vi "XML_MatchLabel.vi"(8 "error in (no error)":errorcluster caption="错误输入（无错误）", 11 "String":string) -> (0 "error out":errorcluster caption="错误输出", 3 "keyValues":T1(array[cluster]))   [LabVIEW 2014]
uses:
  <vilib>/regexp/Match Regular Expression.xnode
panel:
  out "Array":string[](array[string])
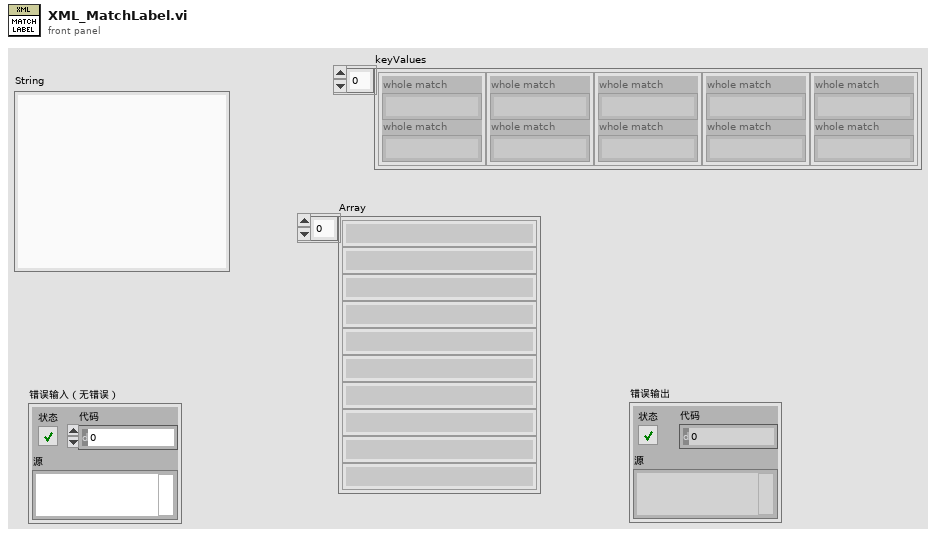
[diagram p1: front panel]
types:
  T1 = cluster{"whole match":string, "whole match":string}[]
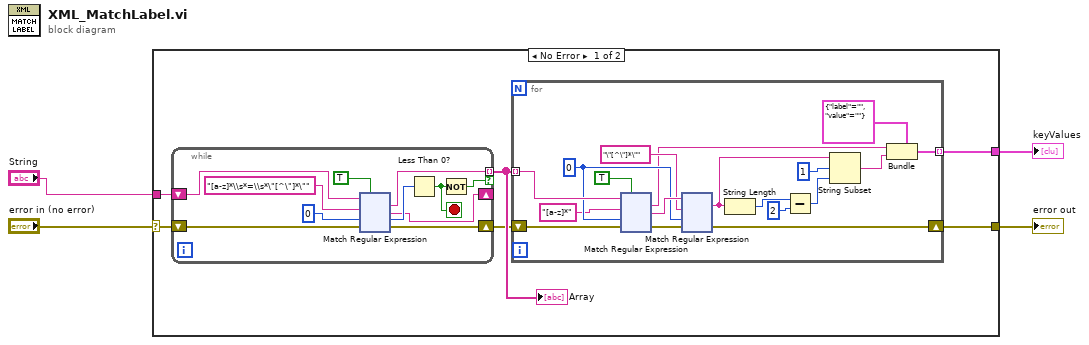
[diagram p0: block diagram]
diagram:
  n1 = case shown="No Error" "error in (no error)" {
    selector: "error in (no error)" -> [w5 w382]
    tunnel: "String" -> [w10 _]
    tunnel: [w7 w382] -> w3
    tunnel: [w6 _] -> w2
    frame No Error {
      n2 = while {
        shift-right: [w262] -> _
        shift-left: w10 -> [w267]
        tunnel: [w264] -> w9 mode=indexing if=w257
        shift-right: [w259] -> w8
        shift-left: w5 -> [w260]
        stop <- w258 stop-if-true
        n3 = xnode "Match Regular Expression"("input string"=w267, "regular expression"="[a-z]*\\s*=\\s*\"[^\"]*\"", "offset (0)"=0, "error in"=w260, "ignore case? (F)"=TRUE) -> ("whole match"=w264:string, "after match"=w262:string, "offset past match"=w263:i32, "error out"=w259:errorcluster)  [unwired: 1 in, 1 out]
        n4 = Less Than 0?(x=w263) -> (x < 0?=w258:bool)
        n5 = Not(x=w258) -> (.not. x?=w257:bool)
      }
      "Array" <- w9
      n6 = for {
        tunnel: w9 -> [w28] mode=indexing
        shift-right: [w20] -> w7
        shift-left: w8 -> [w22]
        tunnel: [w12] -> w6 mode=indexing
        w24 = 0 ("offset (0)")
        n7 = xnode "Match Regular Expression"("input string"=w28, "regular expression"="[a-z]*", "offset (0)"=w24, "error in"=w22, "ignore case? (F)"=TRUE) -> ("whole match"=w14:string, "after match"=w26:string, "error out"=w21:errorcluster)  [unwired: 1 in, 2 out]
        n8 = xnode "Match Regular Expression"("input string"=w26, "regular expression"="\"[^\"]*\"", "offset (0)"=w24, "error in"=w21) -> ("whole match"=w18:string, "error out"=w20:errorcluster)  [unwired: 2 in, 3 out]
        n9 = String Length(string=w18) -> (length=w16:i32)
        n10 = Subtract(x=w16, y=2) -> (x-y=w17:i32)
        n11 = String Subset(string=w18, offset (0)=1, length (rest)=w17) -> (substring=w13:string)
        n12 = Bundle(cluster=cluster{"label":string, "value":string} {"label"="", "value"=""}, "label"=w14, "value"=w13) -> (w12:cluster{"label":string, "value":string})
      }
    }
    frame Error {
    }
  }
  "error out" <- w3
  "keyValues" <- w2
